vi "Host to Target - FPGA.vi"() -> ()   [LabVIEW 2010]
uses:
  <vilib>/rvi/DataTransferAndStorage/Container/XNode/niFpgaContainer.xnode
  <vilib>/rvi/DataTransferAndStorage/Container/Common/niFpgaTransferTypeControl.ctl
  <vilib>/rvi/DataTransferAndStorage/Container/Common/niFpgaContainerMethod.ctl
  <vilib>/rvi/interface/RandomDataEmulation/nirviRandomDataFPGAFIFO.vi
  <vilib>/rvi/interface/RandomDataEmulation/niFpgaRandomDataHandleErrors.vi
panel:
  out "Number of Elements to Read":u32
  in  "FPGA Period(mSec)":u32=100
  out "Timed Out?":bool
  out "Element":i16
  in  "Timeout":i32=100
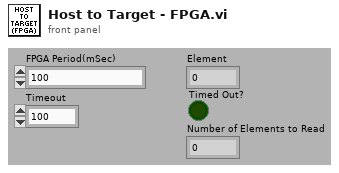
[diagram p1: front panel]
types:
  T1 = typedef "niFpgaContainerMethod.ctl" = enum16{"<none>", "write", "read", "clear", "getNumberOfElementsToWrite", "getNumberOfElementsToRead", "enable", "disable", "flushAndDisable", "getStreamState", "readA", "readB", "dramWrite", "dramWriteWithByteEnables", "dramRequestData", "dramRetrieveData"}
  T2 = typedef "niFpgaTransferTypeControl.ctl" = enum16{"Target-Scoped", "Host to Target - DMA", "Target to Host - DMA", "Peer to Peer Reader", "Peer to Peer Writer", "Bidirectional"}
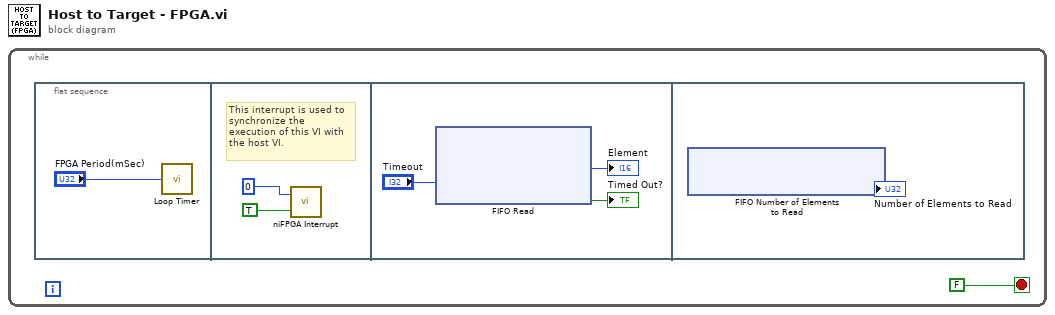
[diagram p0: block diagram]
diagram:
  n1 = while {
    stop <- FALSE stop-if-true
    n2 = flat-sequence {
      frame #0 {
        n3 = call "Loop Timer"("Count(mSec)"="FPGA Period(mSec)") -> ()  [unwired: 1 out]
      }
      frame #1 {
        # "This interrupt is used to synchronize the execution of this VI with the host VI."
        n4 = call <vilib>:"niFPGA Interrupt.vi"("Wait Until Cleared"=TRUE, "IRQ Number"=u8 0) -> ()  [unwired: 1 in]
      }
      frame #2 {
        n5 = xnode ("FIFO Read")("Timeout"="Timeout") -> ("Element"=→"Element":i16, "Timed Out?"=→"Timed Out?":bool)  [unwired: 1 in, 1 out]
      }
      frame #3 {
        n6 = xnode "FIFO Number of Elements to Read"() -> ("Number of Elements to Read"=→"Number of Elements to Read":u32)  [unwired: 1 in, 1 out]
      }
    }
  }
